vi "CVT String StaticRead.vi"(3 "error in (no error)":errorcluster, 5 "Tag Name":string) -> (0 "error out":errorcluster, 1 "Value":string)   [LabVIEW 2016]
uses:
  <vilib>/NI/Current Value Table/DataTypes/String_Static Read.vi
  <vilib>/NI/Current Value Table/Type to Enum.vi
  <vilib>/NI/Current Value Table/DataTypes/String_Type To Enum.vi
  <vilib>/NI/Current Value Table/Memory Block.vi
  <vilib>/NI/Current Value Table/DataTypes/String_Memory Block.vi
  <vilib>/NI/Current Value Table/FGVs/Tag Memory.vi
  <vilib>/NI/Current Value Table/Current Value Table.lvlib
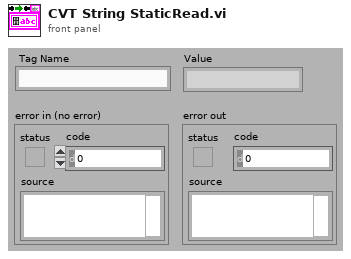
[diagram p1: front panel]
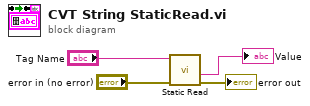
[diagram p0: block diagram]
diagram:
  n1 = call-poly <vilib>:"Static Read.vi"("error in (no error)"="error in (no error)", "Tag Name"="Tag Name") -> ("error out"=→"error out":errorcluster, "Value"=→"Value":string)  [unwired: 8 in]
